vi "Autonomous Independent.vi"() -> ()   [LabVIEW 2019]
doc: "This VI is called when autonomous begins, and will automatically be terminated when autonomous ends. You can carry out timed or sensor driven robot movement independently without needing to return to the caller."
uses:
  <vilib>/Rock Robotics/WPI/ThirdParty/Phoenix-LabVIEW/Pigeon IMU/CTRE_PigeonIMU_TareType.ctl
  <vilib>/Rock Robotics/WPI/Utilities/WPI_GetSetVariantRefNum.vi
  GlobalVariables.vi
  <vilib>/Rock Robotics/WPI/RobotDrive/WPI_RobotDriveArcadeDrive_Standard(NoSaturation).vi
  <vilib>/Utility/file.llb/Read Delimited Spreadsheet (string).vi
  <vilib>/Rock Robotics/Network Tables/NT Read Number.vi
panel:
  in  "Brake Power":dbl=0.025
  in  "Hard coded auto selector":dbl=1.0
  in  "Hard set speed":dbl=0.7
  in  "Shoot, Steal, and Short Line":T1(array[cluster])
  in  "Shoot and Short Line":T1(array[cluster])
  in  "Shoot and Long Line":T1(array[cluster])
  in  "Shoot and Run 3":T1(array[cluster])=[{"Drive "=0.0, "Turn"=0.0, "Wait in ms"=0.0, "Turn?"=FALSE, "Robot States"=enum."ground protect", "Shooter Wheels"=enum."off", "Shooter in range?"=FALSE, "Motion Profile"=FALSE, "Motion Profile File Name"="", "Motion Profile FWD/REV"=FALSE, "Turret Preset"=enum."backward", "Hood Preset"=enum."layup", "Kicker Wheel"=enum."off", "Hopper Wheels"=enum."off"}, {"Drive "=0.0, "Turn"=0.0, "Wait in ms"=1000.0, "Turn?"=FALSE, "Robot States"=enum."ground protect", "Shooter Wheels"=enum."off", "Shooter in range?"=FALSE, "Motion Profile"=FALSE, "Motion Profile File Name"="", "Motion Profile FWD/REV"=FALSE, "Turret Preset"=enum."backward", "Hood Preset"=enum."layup", "Kicker Wheel"=enum."off", "Hopper Wheels"=enum."off"}, {"Drive "=0.0, "Turn"=0.0, "Wait in ms"=4000.0, "Turn?"=FALSE, "Robot States"=enum."ground protect", "Shooter Wheels"=enum."on", "Shooter in range?"=FALSE, "Motion Profile"=FALSE, "Motion Profile File Name"="", "Motion Profile FWD/REV"=FALSE, "Turret Preset"=enum."free track", "Hood Preset"=enum."free track", "Kicker Wheel"=enum."on", "Hopper Wheels"=enum."on"}, {"Drive "=0.0, "Turn"=0.0, "Wait in ms"=0.0, "Turn?"=FALSE, "Robot States"=enum."ground protect", "Shooter Wheels"=enum."off", "Shooter in range?"=FALSE, "Motion Profile"=TRUE, "Motion Profile File Name"="shootrun3a", "Motion Profile FWD/REV"=TRUE, "Turret Preset"=enum."backward", "Hood Preset"=enum."layup", "Kicker Wheel"=enum."off", "Hopper Wheels"=enum."off"}]
  in  "Shoot and Trench 6":T1(array[cluster])=[{"Drive "=0.0, "Turn"=0.0, "Wait in ms"=0.0, "Turn?"=FALSE, "Robot States"=enum."ground protect", "Shooter Wheels"=enum."off", "Shooter in range?"=FALSE, "Motion Profile"=FALSE, "Motion Profile File Name"="", "Motion Profile FWD/REV"=FALSE, "Turret Preset"=enum."backward", "Hood Preset"=enum."layup", "Kicker Wheel"=enum."off", "Hopper Wheels"=enum."off"}, {"Drive "=0.0, "Turn"=0.0, "Wait in ms"=1000.0, "Turn?"=FALSE, "Robot States"=enum."ground protect", "Shooter Wheels"=enum."on", "Shooter in range?"=FALSE, "Motion Profile"=FALSE, "Motion Profile File Name"="", "Motion Profile FWD/REV"=FALSE, "Turret Preset"=enum."backward", "Hood Preset"=enum."layup", "Kicker Wheel"=enum."off", "Hopper Wheels"=enum."off"}, {"Drive "=0.0, "Turn"=0.0, "Wait in ms"=3500.0, "Turn?"=FALSE, "Robot States"=enum."ground protect", "Shooter Wheels"=enum."on", "Shooter in range?"=FALSE, "Motion Profile"=FALSE, "Motion Profile File Name"="", "Motion Profile FWD/REV"=FALSE, "Turret Preset"=enum."free track", "Hood Preset"=enum."free track", "Kicker Wheel"=enum."on", "Hopper Wheels"=enum."on"}, {"Drive "=0.0, "Turn"=0.0, "Wait in ms"=0.0, "Turn?"=FALSE, "Robot States"=enum."ground pickup", "Shooter Wheels"=enum."off", "Shooter in range?"=FALSE, "Motion Profile"=TRUE, "Motion Profile File Name"="shoottrench6a", "Motion Profile FWD/REV"=FALSE, "Turret Preset"=enum."backward", "Hood Preset"=enum."free track", "Kicker Wheel"=enum."on", "Hopper Wheels"=enum."on"}, {"Drive "=0.0, "Turn"=0.0, "Wait in ms"=0.0, "Turn?"=FALSE, "Robot States"=enum."ground protect", "Shooter Wheels"=enum."on", "Shooter in range?"=FALSE, "Motion Profile"=FALSE, "Motion Profile File Name"="shoottrench6b", "Motion Profile FWD/REV"=TRUE, "Turret Preset"=enum."free track", "Hood Preset"=enum."free track", "Kicker Wheel"=enum."off", "Hopper Wheels"=enum."off"}, {"Drive "=0.0, "Turn"=0.0, "Wait in ms"=5000.0, "Turn?"=FALSE, "Robot States"=enum."ground protect", "Shooter Wheels"=enum."on", "Shooter in range?"=FALSE, "Motion Profile"=FALSE, "Motion Profile File Name"="", "Motion Profile FWD/REV"=FALSE, "Turret Preset"=enum."free track", "Hood Preset"=enum."free track", "Kicker Wheel"=enum."on", "Hopper Wheels"=enum."on"}]
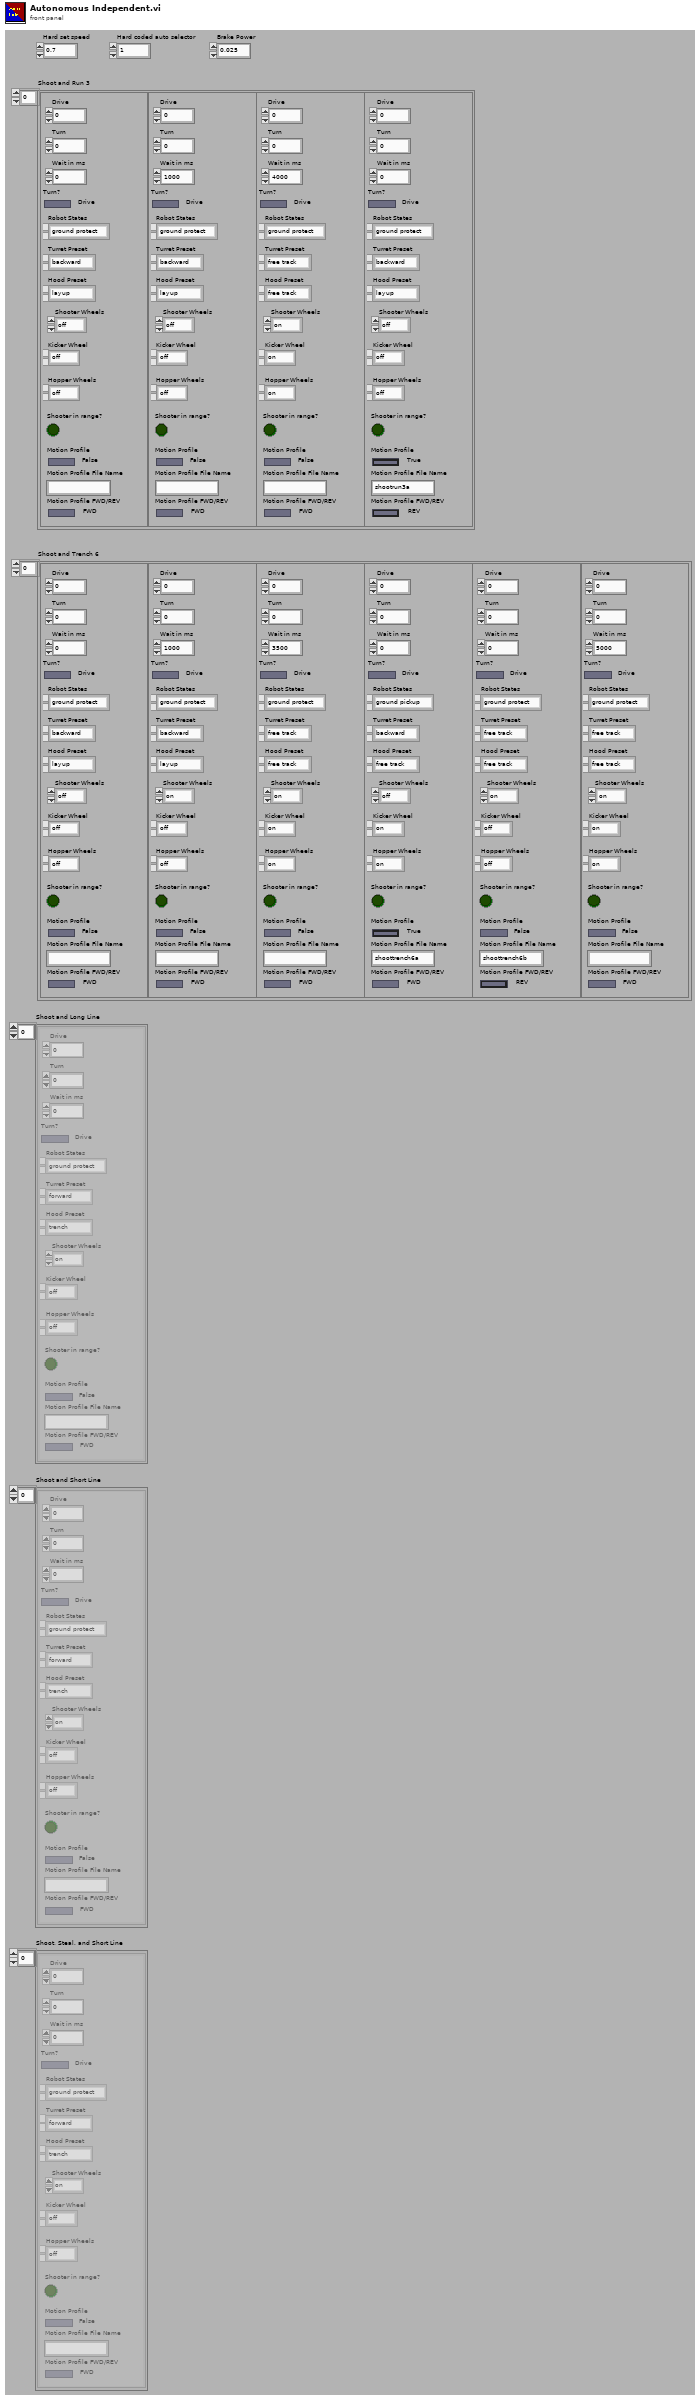
[diagram p1: front panel]
types:
  T1 = cluster{"Drive ":dbl, "Turn":dbl, "Wait in ms":dbl, "Turn?":bool, "Robot States":enum16{"ground protect", "ground pickup", "control panel", "shooting", "climb", "unjam", "intake shoot"}, "Shooter Wheels":enum16{"on", "off"}, "Shooter in range?":bool, "Motion Profile":bool, "Motion Profile File Name":string, "Motion Profile FWD/REV":bool, "Turret Preset":enum16{"free track", "forward", "backward"}, "Hood Preset":enum16{"trench", "layup", "free track"}, "Kicker Wheel":enum16{"on", "off", "reverse"}, "Hopper Wheels":enum16{"on", "off"}}[]
  T2 = typedef "CTRE_PigeonIMU_TareType.ctl" = u8
  T3 = enum16{"Shoot and Run 3", "Shoot and Trench 6", "Shoot and Long Line", "Shoot and Short Line", "Shoot, Steal, and Short Line"}
  T4 = typedef "CTRE_PigeonIMU_DeviceRef.ctl" = cluster{"DeviceStatus":errorcluster, "Device Number":u8, "Type":T5, "Device ID":u32, "Handle":u64, "UsageFrame":u32, "Library Path":path}
  T5 = typedef "CTRE_PigeonIMU_ConnectionType.ctl" = u32
  T6 = typedef "WPI_RobotDriveDevRef.ctl" = cluster{"DevStatus":errorcluster, "Motors[]":T7[], "Square Inputs":bool, "Max Output":dbl}
  T7 = typedef "WPI_MotorControlDeviceRef.ctl" = cluster{"DeviceStatus":errorcluster, "Type":T8, "PWM":cluster{"PWM Channel":T9, "DeadBand":T10}, "CAN":cluster{"Device Number":u8, "SetOutput VI Ref":variant, "GetOutput VI Ref":variant, "Enable VI Ref":variant, "Disable VI Ref":variant, "Data":variant}, "Invert":bool, "DIO PWM":cluster{"PWM \"Enable\" Channel":T9, "DIOChannel":T11, "PWM Rate":dbl}}
  T8 = typedef "WPI_MotorControlType.ctl" = enum16{"PWM", "CAN", "DIO PWM"}
  T9 = typedef "FPGA_DIOPWMChannel.ctl" = enum8{"PWM 0", "PWM 1", "PWM 2", "PWM 3", "PWM 4", "PWM 5", "PWM 6", "PWM 7", "PWM 8", "PWM 9", "PWM MXP 0", "PWM MXP 1", "PWM MXP 2", "PWM MXP 3", "PWM MXP 4", "PWM MXP 5", "PWM MXP 6", "PWM MXP 7", "PWM MXP 8", "PWM MXP 9", "Invalid"}
  T10 = typedef "WPI_PWMDeadband.ctl" = cluster{"Name":string, "maxPositivePwm":i32, "minPositivePwm":i32, "centerPwm":i32, "maxNegativePwm":i32, "minNegativePwm":i32, "angularRange":u16}
  T11 = typedef "FPGA_DIOChannel.ctl" = enum8{"DIO 0", "DIO 1", "DIO 2", "DIO 3", "DIO 4", "DIO 5", "DIO 6", "DIO 7", "DIO 8", "DIO 9", "DIO MXP 0", "DIO MXP 1", "DIO MXP 2", "DIO MXP 3", "DIO MXP 4", "DIO MXP 5", "DIO MXP 6", "DIO MXP 7", "DIO MXP 8", "DIO MXP 9", "DIO MXP 10", "DIO MXP 11", "DIO MXP 12", "DIO MXP 13", "DIO MXP 14", "DIO MXP 15", "SPI Port CS1", "SPI Port CS2", "SPI Port CS3", "SPI Port MISO", "SPI Port MOSI", "Invalid"}
  T12 = enum16{"ground protect", "ground pickup", "control panel", "shooting", "climb", "unjam", "intake shoot"}
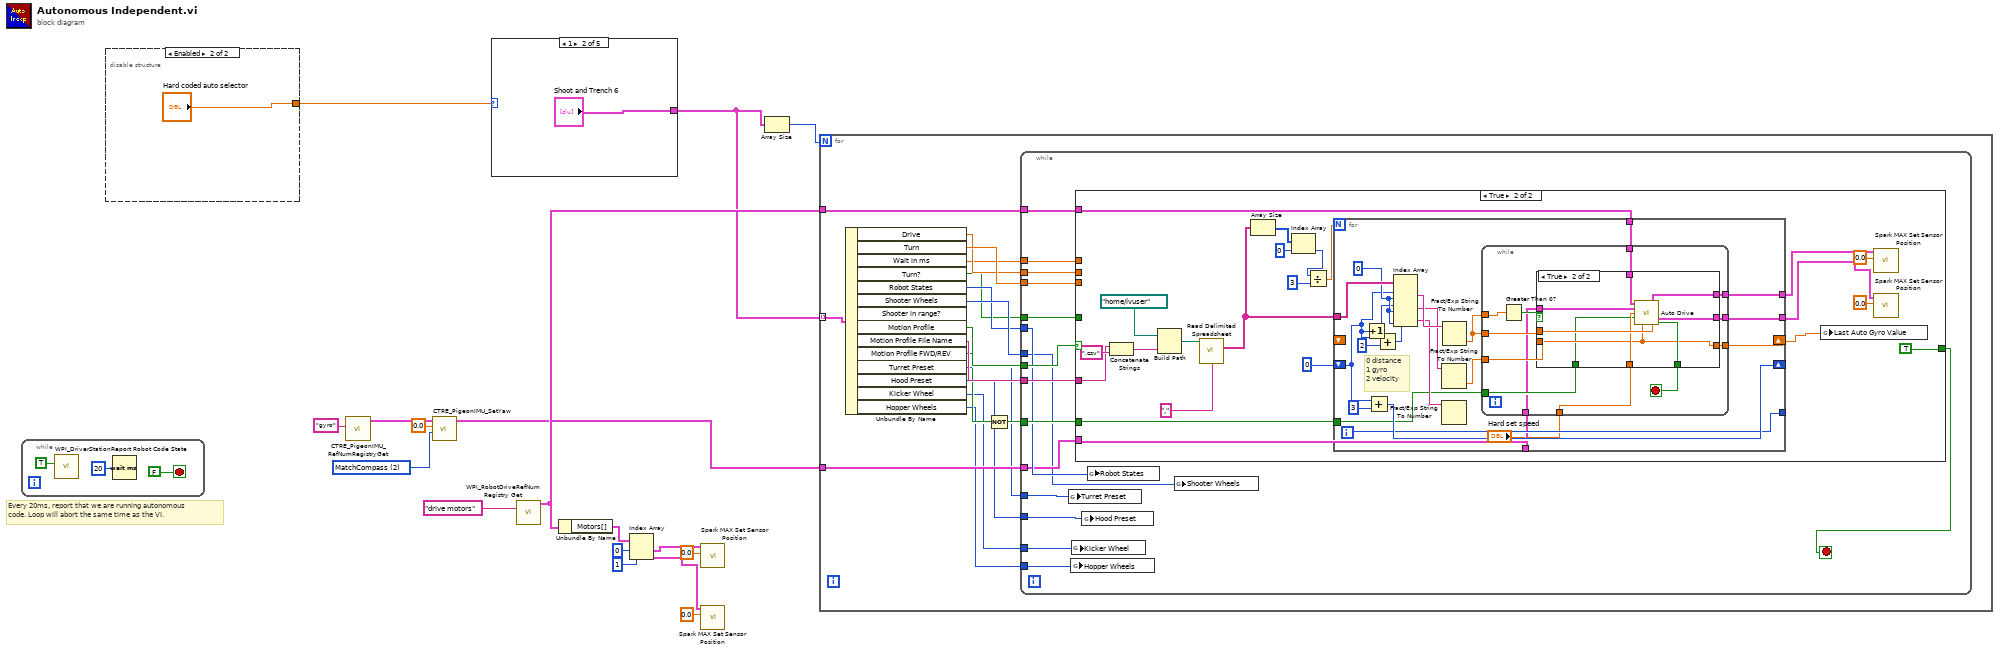
[diagram p0: block diagram]
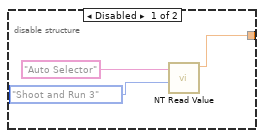
[diagram p2: hidden frame]
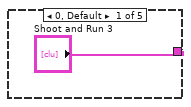
[diagram p3: hidden frame]
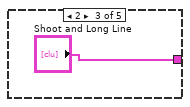
[diagram p4: hidden frame]
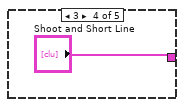
[diagram p5: hidden frame]
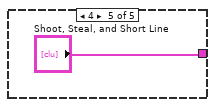
[diagram p6: hidden frame]
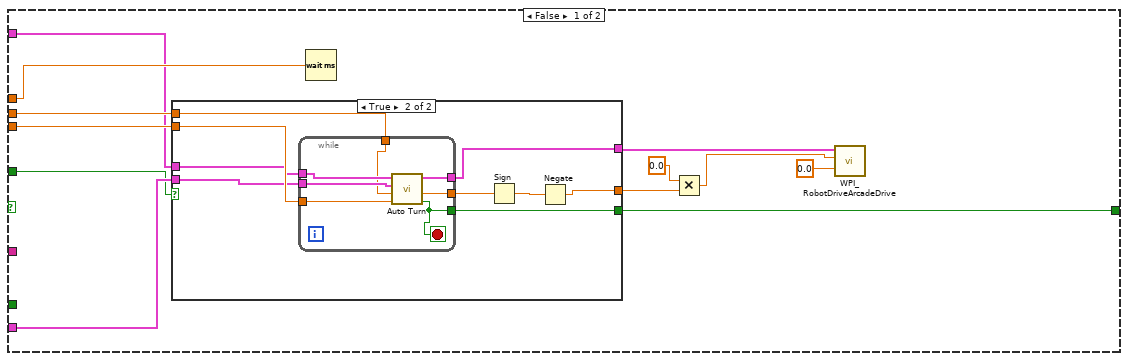
[diagram p7: hidden frame]
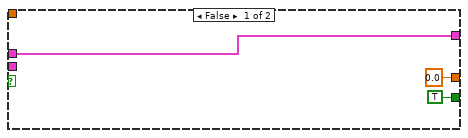
[diagram p8: hidden frame]
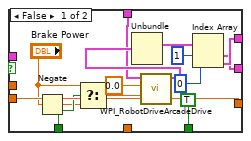
[diagram p9: hidden frame]
diagram:
  w5 = T2 2 items=["SetValue"=0, "AddOffset"=1, "MatchCompass"=2, "SetOffset"=255] ("TareType (SetValue)")
  # "Every 20ms, report that we are running autonomous\ncode. Loop will abort the same time as the VI."
  n1 = while {
    stop <- FALSE stop-if-true
    n2 = call <vilib>:"WPI_DriverStationReport Robot Code State.vi"("Autonomous"=TRUE) -> ()  [unwired: 10 in, 1 out]
    n3 = Wait (ms)(milliseconds to wait=u32 20) -> ()  [unwired: 1 out]
  }
  n4 = disable-structure shown="Enabled" {
    disable-tunnel: [w22 "Hard coded auto selector"] -> w3
    frame Disabled {
      n5 = call-poly <vilib>:"NT Read Value.vi"("Default Value"=T3."Shoot and Run 3", "Name"="Auto Selector") -> ("Numeric"=w22:dbl)  [unwired: 8 in, 1 out]
    }
    frame Enabled {
    }
  }
  n6 = call <vilib>:"CTRE_PigeonIMU_RefNumRegistryGet.vi"("refnum name"="gyro") -> ("PigeonIMUDevRef"=w8:T4)  [unwired: 9 in, 1 out]
  n7 = call <vilib>:"CTRE_PigeonIMU_SetYaw.vi"("TareType (SetValue)"=w5, "Value"=0.0, "PigeonIMUDevRef"=w8) -> ("PigeonIMUDevRef"=w7:T4)  [unwired: 7 in, 1 out]
  n8 = case shown="1" w3 {
    tunnel: ["Shoot and Run 3" "Shoot and Trench 6" "Shoot and Long Line" "Shoot and Short Line" "Shoot, Steal, and Short Line"] -> w2
    frame 0, Default {
    }
    frame 1 {
    }
    frame 2 {
    }
    frame 3 {
    }
    frame 4 {
    }
  }
  n9 = call <vilib>:"WPI_RobotDriveRefNum Registry Get.vi"("refnum name"="drive motors") -> ("RobotDriveDevRef"=w9:T6)  [unwired: 9 in, 1 out]
  n10 = Unbundle By Name(w9) -> ("Motors[]"=w11:T7[])
  n11 = Index Array(array=w11, index #1=0 ("index"), index #2=1 ("index")) -> (element #1=w13:T7, element #2=w17:T7)
  n12 = call <vilib>:"Spark MAX Set Sensor Position.vi"("Position"=0.0, "MotorControlDeviceRef"=w13) -> ()  [unwired: 8 in, 2 out]
  n13 = call <vilib>:"Spark MAX Set Sensor Position.vi"("Position"=0.0, "MotorControlDeviceRef"=w17) -> ()  [unwired: 8 in, 2 out]
  n14 = Array Size(array=w2) -> (size(s)=w1:i32)
  n15 = for {
    N: w1 -> [_]
    tunnel: w2 -> [w38] mode=indexing
    tunnel: w9 -> [w36]
    tunnel: w7 -> [w35]
    n16 = Unbundle By Name(w38) -> ("Drive"=w44:dbl, "Turn"=w45:dbl, "Wait in ms"=w39:dbl, "Turn?"=w34:bool, "Robot States"=w42:T12, "Shooter Wheels"=w43:enum16{"on", "off"}, "Motion Profile"=w46:bool, "Motion Profile File Name"=w41:string, "Motion Profile FWD/REV"=w37:bool, "Turret Preset"=w33:enum16{"free track", "forward", "backward"}, "Hood Preset"=w32:enum16{"trench", "layup", "free track"}, "Kicker Wheel"=w31:enum16{"on", "off", "reverse"}, "Hopper Wheels"=w30:enum16{"on", "off"})  [unwired: 1 out]
    n17 = Not(x=w37) -> (.not. x?=w40:bool)
    n18 = while {
      tunnel: w46 -> [w56]
      tunnel: w45 -> [w62]
      tunnel: w44 -> [w61]
      tunnel: w43 -> [w49]
      tunnel: w42 -> [w54]
      tunnel: w41 -> [w59]
      tunnel: w40 -> [w58]
      tunnel: w39 -> [w57]
      tunnel: w36 -> [w55]
      tunnel: w35 -> [w53]
      tunnel: w34 -> [w52]
      tunnel: w33 -> [w51]
      tunnel: w32 -> [w50]
      tunnel: w31 -> [w48]
      tunnel: w30 -> [w47]
      stop <- w60 stop-if-true
      n19 = global write "GlobalVariables.vi" "Turret Preset"(w51) -> ()
      n20 = global write "GlobalVariables.vi" "Hopper Wheels"(w47) -> ()
      n21 = global write "GlobalVariables.vi" "Kicker Wheel"(w48) -> ()
      n22 = case shown="True" w56 {
        tunnel: w62 -> [w74 _]
        tunnel: w61 -> [w73 _]
        tunnel: [w72 TRUE ("In Range?")] -> w60
        tunnel: w59 -> [_ w94]
        tunnel: w58 -> [_ w102]
        tunnel: w57 -> [w66 _]
        tunnel: w55 -> [w65 w96]
        tunnel: w53 -> [w64 w95]
        tunnel: w52 -> [w63 _]
        frame False {
          n23 = case shown="True" w63 {
            tunnel: w74 -> [_ w85]
            tunnel: w73 -> [_ w86]
            tunnel: [TRUE ("In Range?") w84] -> w72
            tunnel: [w77 w83] -> w67
            tunnel: [0.0 w80] -> w69
            tunnel: w65 -> [w77 w79]
            tunnel: w64 -> [_ w78]
            frame False {
            }
            frame True {
              n24 = while {
                tunnel: w86 -> [w88]
                tunnel: w85 -> [w87]
                tunnel: [w91] -> w84
                tunnel: [w92] -> w82
                tunnel: [w93] -> w83
                tunnel: w79 -> [w90]
                tunnel: w78 -> [w89]
                stop <- w91 stop-if-true
                n25 = call "Auto Turn.vi"("X setpoint"=w87, "Y axis value"=w88, "PigeonIMUDevRef"=w89, "Drive Dev Ref in"=w90) -> ("In Range?"=w91:bool, "X axis value out"=w92:dbl, "Drive Dev Ref out"=w93:T6)  [unwired: 4 in, 1 out]
              }
              n26 = Sign(1:w82) -> (0:w81:dbl)
              n27 = Negate(x=w81) -> (-x=w80:dbl)
            }
          }
          n28 = Wait (ms)(milliseconds to wait=w66) -> ()  [unwired: 1 out]
          n29 = Multiply(x=0.0, y=w69) -> (x*y=w68:dbl)
          n30 = call-poly <vilib>:"WPI_RobotDriveArcadeDrive.vi"("Y axis value"=0.0, "X axis value"=w68, "RobotDriveDevRef"=w67) -> ()  [unwired: 6 in, 3 out]
        }
        frame True {
          n31 = Concatenate Strings(w94, ".csv" ("string")) -> (w105:string)
          n32 = Build Path(base path=path "/home/lvuser" ("file path (dialog if empty)"), name or relative path=w105) -> (appended path=w106:path)
          n33 = call-poly <vilib>:"Read Delimited Spreadsheet.vi"("file path (dialog if empty)"=w106, "delimiter (\\t)"=",") -> ("all rows"=w103:string[][])  [unwired: 8 in, 5 out]
          n34 = Array Size(array=w103) -> (size(s)=w114:i32[])
          n35 = Index Array(array=w114, index=0) -> (element=w110:i32)
          n36 = Divide(x=w110, y=3) -> (x/y=w108:dbl)
          n37 = for {
            N: w108 -> [_]
            shift-right: [w135] -> _
            shift-left: 0 -> [w128]
            tunnel: w103 -> [w132]
            tunnel: w102 -> [w124]
            tunnel: [w123] -> _
            shift-right: [w122] -> w97
            shift-left: _ -> [_]
            tunnel: [w121] -> w98
            tunnel: [w120] -> w99
            tunnel: w96 -> [w119]
            tunnel: w95 -> [w118]
            i -> [w123]
            w129 = 0 ("index (row)")
            # "0 distance\n1 gyro\n2 velocity"
            n38 = Increment(x=w128) -> (x+1=w127:i32)
            n39 = Add(x=w128, y=3) -> (x+y=w135:i32)
            n40 = Add(x=w128, y=2) -> (x+y=w126:i32)
            n41 = Index Array(array=w132, index (row) #1=w128, index (col) #1=w129, index (row) #2=w127, index (col) #2=w129, index (row) #3=w126, index (col) #3=w129) -> (element #1=w131:string, element #2=w130:string, element #3=w125:string)
            n42 = Fract/Exp String To Number(string=w130) -> (number=w116:dbl)  [unwired: 3 in, 1 out]
            n43 = Fract/Exp String To Number(string=w125) -> ()  [unwired: 3 in, 2 out]
            n44 = Fract/Exp String To Number(string=w131) -> (number=w133:dbl)  [unwired: 3 in, 1 out]
            n45 = while {
              tunnel: w133 -> [w140]
              tunnel: w116 -> [w141]
              tunnel: w133 -> [w146]
              tunnel: "Hard set speed" -> [w145]
              tunnel: w124 -> [w139]
              tunnel: [w144] -> w122
              tunnel: [w143] -> w121
              tunnel: [w142] -> w120
              tunnel: w119 -> [w138]
              tunnel: w118 -> [w137]
              stop <- w148 stop-if-true
              n46 = Greater Than 0?(x=w146) -> (x > 0?=w147:bool)
              n47 = case shown="True" w147 {
                tunnel: [TRUE ("In Range?") w171] -> w148
                tunnel: w140 -> [_ w170]
                tunnel: w141 -> [w161 w168]
                tunnel: w145 -> [_ w169]
                tunnel: [w161 w168] -> w144
                tunnel: [w155 w167] -> w143
                tunnel: [w156 w166] -> w142
                tunnel: w139 -> [w151 w165]
                tunnel: w138 -> [w154 w164]
                tunnel: w137 -> [_ w163]
                frame False {
                  n48 = Negate(x="Brake Power") -> (-x=w149:dbl)
                  n49 = Select(t="Brake Power", s=w151, f=w149) -> (s? t:f=w153:dbl)
                  n50 = call-poly <vilib>:"WPI_RobotDriveArcadeDrive.vi"("Y axis value"=w153, "X axis value"=0.0, "RobotDriveDevRef"=w154) -> ("RobotDriveDevRef"=w160:T6)  [unwired: 6 in, 2 out]
                  n51 = Unbundle(w160) -> ("Motors[]"=w159:T7[])  [unwired: 3 out]
                  n52 = Index Array(array=w159, index #1=1 ("index"), index #2=0 ("index")) -> (element #1=w155:T7, element #2=w156:T7)
                }
                frame True {
                  n53 = call "Auto Drive.vi"("Drive Dev Ref in"=w164, "PigeonIMUDevRef in"=w163, "Y Input Speed"=w169, "FWD/REV"=w165, "X setpoint"=w168, "Y setpoint"=w170) -> ("Left Drive Encoder Out"=w166:T7, "Right Drive Encoder Out"=w167:T7, "In Range?"=w171:bool)  [unwired: 4 in, 3 out]
                }
              }
            }
          }
          n54 = global write "GlobalVariables.vi" "Last Auto Gyro Value"(w97) -> ()
          n55 = call <vilib>:"Spark MAX Set Sensor Position.vi"("Position"=0.0, "MotorControlDeviceRef"=w99) -> ()  [unwired: 8 in, 2 out]
          n56 = call <vilib>:"Spark MAX Set Sensor Position.vi"("Position"=0.0, "MotorControlDeviceRef"=w98) -> ()  [unwired: 8 in, 2 out]
        }
      }
      n57 = global write "GlobalVariables.vi" "Hood Preset"(w50) -> ()
      n58 = global write "GlobalVariables.vi" "Robot States"(w54) -> ()
      n59 = global write "GlobalVariables.vi" "Shooter Wheels"(w49) -> ()
    }
  }
